vi "ATS_Specs_Selection.vi"(9 "ID":i32, 10 "Device":i32=-1, 11 "ATS_Spec_Selector":T4) -> (0 "Disabled_Item":i32[](array[numeric]), 1 "Possible_Item":string[](array[string]), 2 "All_Item":string[](array[string]), 3 "Selection":string, 4 "Other":cluster{"ValueName":string, "Value":u32}, 5 "Specifications":T5={"ClckSource"={"Internal"=FALSE, "External"=FALSE, "Medium Ext."=FALSE, "Slow Ext."=FALSE, "Ext. AC"=FALSE, "Ext. DC"=FALSE, "Ext. (PLL)"=FALSE}, "ClckRate"={"1 kS/s"=FALSE, "2 kS/s"=FALSE, "5 kS/s"=FALSE, "10 kS/s"=FALSE, "20 kS/s"=FALSE, "50 kS/s"=FALSE, "100 kS/s"=FALSE, "200 kS/s"=FALSE, "500 kS/s"=FALSE, "1 MS/s"=FALSE, "2 MS/s"=FALSE, "5 MS/s"=FALSE, "10 MS/s"=FALSE, "20 MS/s"=FALSE, "25 MS/s"=FALSE, "50 MS/s"=FALSE, "100 MS/s"=FALSE, "125 MS/s"=FALSE, "160 MS/s"=FALSE, "180 MS/s"=FALSE, "200 MS/s"=FALSE, "250 MS/s"=FALSE, "500 MS/s"=FALSE, "1 GS/s"=FALSE}, "ClckEdge"={"Rising"=FALSE, "Falling"=FALSE}, "InputCoupling"={"AC"=FALSE, "DC"=FALSE}, "InputRange"={"20mV"=FALSE, "40mV"=FALSE, "50mV"=FALSE, "80mV"=FALSE, "100mV"=FALSE, "200mV"=FALSE, "400mV"=FALSE, "500mV"=FALSE, "800mV"=FALSE, "1 V"=FALSE, "2 V"=FALSE, "4 V"=FALSE, "5 V"=FALSE, "8 V"=FALSE, "10 V"=FALSE, "16 V"=FALSE, "20 V"=FALSE, "40 V"=FALSE, "HiFi"=FALSE, "1.25 V"=FALSE}, "Impedance"={"1M ohms"=FALSE, "50 ohms"=FALSE, "300 ohms"=FALSE}, "Bandwidth"={"Full"=FALSE, "Reduce"=FALSE}, "RangeLim(50)"="", "AsyncDMA"={"OnBoard"=FALSE, "FPGA"=FALSE}, "Memory"={"VerifMem"=FALSE, "HighMem"=FALSE, "Combine"=FALSE, "HighRecord"=FALSE}, "ExtTrigCoupling"={"AC"=FALSE, "DC"=FALSE}, "ExtTrigRange"={"1 V"=FALSE, "5 V"=FALSE, "\nTTL"=FALSE}, "AUX_IO_Trig"={"Trig_Out"=FALSE, "Trig_In"=FALSE}, "AUX_IO_Slope"={"Rising"=FALSE, "Falling"=FALSE}, "MaxPretrig"={"MEM"=0, "FIFO"=0}, "AUX_I/O_Trig"={"OUT_Trigger"=FALSE, "OUT_PACER"=FALSE, "OUT_BUSY"=FALSE, "OUT_CLOCK"=FALSE, "OUT_RESERVED"=FALSE, "OUT_CAPTURE_ALMOST_DONE"=FALSE, "OUT_AUXILIARY"=FALSE, "OUT_SERIAL_DATA"=FALSE, "IN_TRIGGER_ENABLE"=FALSE, "IN_DIGITAL_TRIGGER"=FALSE, "IN_GATE"=FALSE, "IN_CAPTURE_ON_DEMAND"=FALSE, "IN_RESET_TIMESTAMP"=FALSE, "IN_SLOW_EXTERNAL_CLOCK"=FALSE, "INPUT_AUXILIARY"=FALSE, "INPUT_SERIAL_DATA"=FALSE}, "ChannelsPerBoard"=2}, 7 "Device_Name":string)   [LabVIEW 2015]
doc: "_____AlazarTech, Scope_____\n\nExtract the Selected Specifications of the ID Board and create a text array of All, Possible and Disable item.\n\nIf Device = -1 than use the ID input otherwise select the device.\n\nOutput:\n- Selection: option read\n-All_Item: all specifications array\n-Possible_Item: available specification array\n-Disabled_Item: array of item number which are not available."
uses:
  ATS_ctl/ATS_Global_Specs_Ctrl.ctl
  ATS_ctl/ATS_Spec_Selector.ctl
  ATS_ctl/ATS_TriggerEngine_4Ch.ctl
  ATS_ctl/ATS_TriggerSource_4Ch.ctl
  ATS_ctl/TriggerEngine.ctl
  ATS_ctl/ATS_Global_Ctrl.ctl
  ATS_ctl/ATS_Cards_GBL.vi
panel:
  in  "TrigEngine":T1
  in  "TriggerEngine_4Ch":T2
  out "Device_ID":string
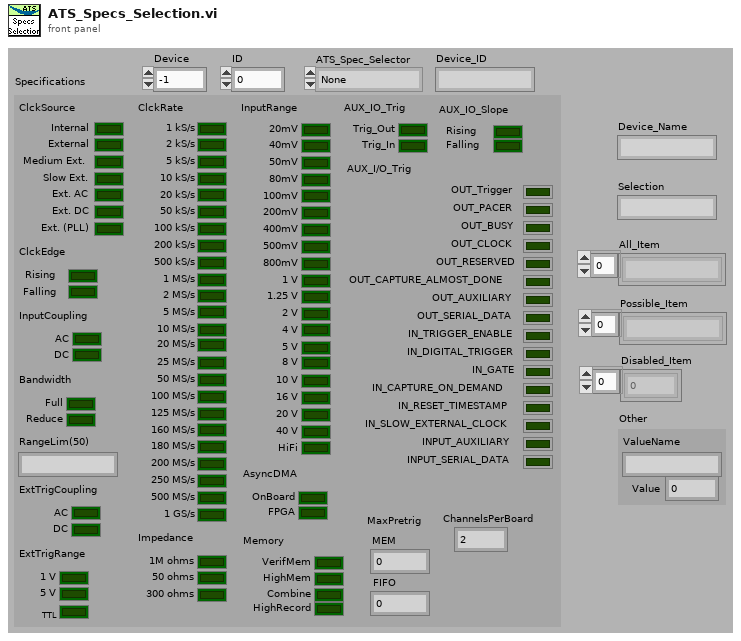
[diagram p1: front panel]
types:
  T1 = typedef "TriggerEngine.ctl" = cluster{"Source":enum32{"Chan_A", "Chan_B", "External", "Disable"}, "Slope":enum32{"Positive", "Negative"}, "Level":u32}
  T2 = typedef "ATS_TriggerEngine_4Ch.ctl" = cluster{"Source":T3, "Slope":enum32{"Positive", "Negative"}, "Level":u32}
  T3 = typedef "ATS_TriggerSource_4Ch.ctl" = enum32{"Chan_A", "Chan_B", "External", "Disable", "Chan_C", "Chan_D"}
  T4 = typedef "ATS_Spec_Selector.ctl" = enum16{"None", "ClckSource", "ClckEdge", "ClckRate", "InputRange", "InputCoupling", "Impedance", "Bandwidth", "AsyncDMA", "Memory", "ExtTrigCoupling", "ExtTrigRange", "AUX_IO_Trig", "AUX_IO_Slope", "Trigger_Source"}
  T5 = typedef "ATS_Global_Specs_Ctrl.ctl" = cluster{"ClckSource":cluster{"Internal":bool, "External":bool, "Medium Ext.":bool, "Slow Ext.":bool, "Ext. AC":bool, "Ext. DC":bool, "Ext. (PLL)":bool}, "ClckRate":cluster{"1 kS/s":bool, "2 kS/s":bool, "5 kS/s":bool, "10 kS/s":bool, "20 kS/s":bool, "50 kS/s":bool, "100 kS/s":bool, "200 kS/s":bool, "500 kS/s":bool, "1 MS/s":bool, "2 MS/s":bool, "5 MS/s":bool, "10 MS/s":bool, "20 MS/s":bool, "25 MS/s":bool, "50 MS/s":bool, "100 MS/s":bool, "125 MS/s":bool, "160 MS/s":bool, "180 MS/s":bool, "200 MS/s":bool, "250 MS/s":bool, "500 MS/s":bool, "1 GS/s":bool}, "ClckEdge":cluster{"Rising":bool, "Falling":bool}, "InputCoupling":cluster{"AC":bool, "DC":bool}, "InputRange":cluster{"20mV":bool, "40mV":bool, "50mV":bool, "80mV":bool, "100mV":bool, "200mV":bool, "400mV":bool, "500mV":bool, "800mV":bool, "1 V":bool, "2 V":bool, "4 V":bool, "5 V":bool, "8 V":bool, "10 V":bool, "16 V":bool, "20 V":bool, "40 V":bool, "HiFi":bool, "1.25 V":bool}, "Impedance":cluster{"1M ohms":bool, "50 ohms":bool, "300 ohms":bool}, "Bandwidth":cluster{"Full":bool, "Reduce":bool}, "RangeLim(50)":string, "AsyncDMA":cluster{"OnBoard":bool, "FPGA":bool}, "Memory":cluster{"VerifMem":bool, "HighMem":bool, "Combine":bool, "HighRecord":bool}, "ExtTrigCoupling":cluster{"AC":bool, "DC":bool}, "ExtTrigRange":cluster{"1 V":bool, "5 V":bool, "\nTTL":bool}, "AUX_IO_Trig":cluster{"Trig_Out":bool, "Trig_In":bool}, "AUX_IO_Slope":cluster{"Rising":bool, "Falling":bool}, "MaxPretrig":cluster{"MEM":u32, "FIFO":u32}, "AUX_I/O_Trig":cluster{"OUT_Trigger":bool, "OUT_PACER":bool, "OUT_BUSY":bool, "OUT_CLOCK":bool, "OUT_RESERVED":bool, "OUT_CAPTURE_ALMOST_DONE":bool, "OUT_AUXILIARY":bool, "OUT_SERIAL_DATA":bool, "IN_TRIGGER_ENABLE":bool, "IN_DIGITAL_TRIGGER":bool, "IN_GATE":bool, "IN_CAPTURE_ON_DEMAND":bool, "IN_RESET_TIMESTAMP":bool, "IN_SLOW_EXTERNAL_CLOCK":bool, "INPUT_AUXILIARY":bool, "INPUT_SERIAL_DATA":bool}, "ChannelsPerBoard":u8}
  T6 = typedef "ATS_Global_Ctrl.ctl" = enum16{"Init_Device", "Clear_ALL", "Set", "Get"}
  T7 = typedef "Device_Info.ctl" = cluster{"Handle":u32, "Board":string, "CPLD":string, "MemorySize":u32, "SampleSize":u8, "ID":i32, "High_Memory":bool, "Chan/Board":u8}
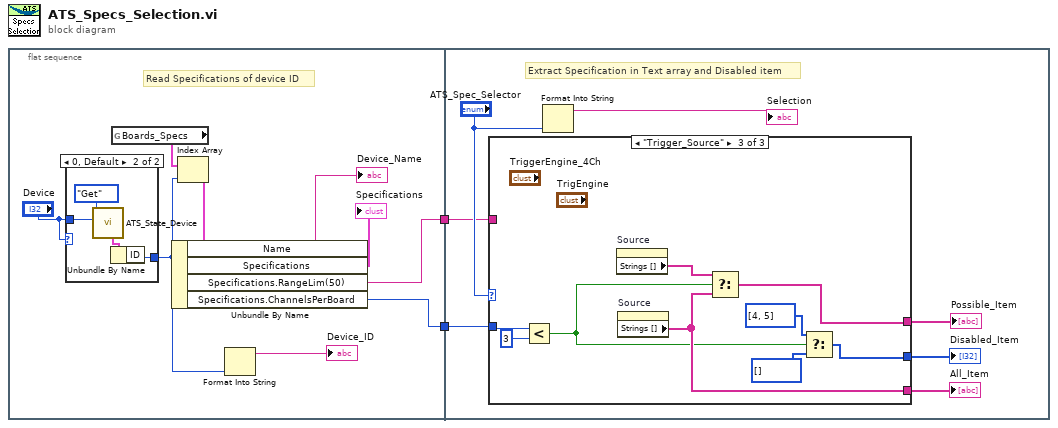
[diagram p0: block diagram]
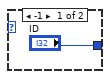
[diagram p2: hidden frame]
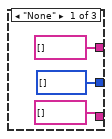
[diagram p3: hidden frame]
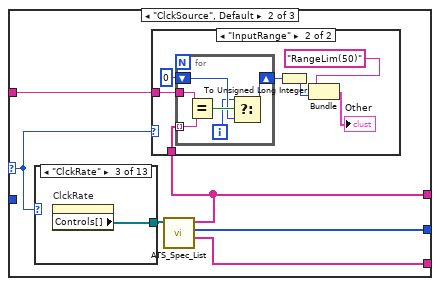
[diagram p4: hidden frame]
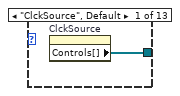
[diagram p6: hidden frame]
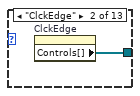
[diagram p7: hidden frame]
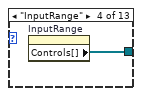
[diagram p8: hidden frame]
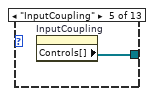
[diagram p9: hidden frame]
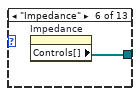
[diagram p10: hidden frame]
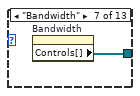
[diagram p11: hidden frame]
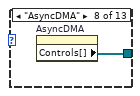
[diagram p12: hidden frame]
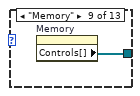
[diagram p13: hidden frame]
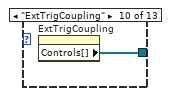
[diagram p14: hidden frame]
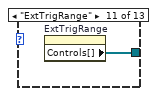
[diagram p15: hidden frame]
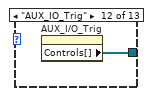
[diagram p16: hidden frame]
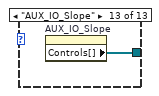
[diagram p17: hidden frame]
diagram:
  n1 = flat-sequence {
    tunnel: [w7] -> w2
    tunnel: [w3] -> w1
    tunnel: w2 -> [w21]
    tunnel: w1 -> [w17]
    frame #0 {
      # "Read Specifications of device ID"
      n2 = case shown="0, Default" "Device" {
        tunnel: "Device" -> [_ w15]
        tunnel: ["ID" w13] -> w5
        frame -1 {
        }
        frame 0, Default {
          n3 = call "ATS_State_Device.vi"("DeviceIn"=w15, "ATS_GBL_Ctrl"=ATS_Global_Ctrl."Get") -> ("DevInfo_Out"=w14:T7)  [unwired: 4 in, 5 out]
          n4 = Unbundle By Name(w14) -> ("ID"=w13:i32)
        }
      }
      n5 = global read "ATS_Cards_GBL.vi" "Boards_Specs"() -> (w4:cluster{"Name":string, "Specifications":T5}[])
      n6 = Index Array(array=w4, index=w5) -> (element=w11:cluster{"Name":string, "Specifications":T5})
      n7 = Unbundle By Name(w11) -> ("Name"=→"Device_Name":string, "Specifications"=→"Specifications":T5, "Specifications.RangeLim(50)"=w7:string, "Specifications.ChannelsPerBoard"=w3:u8)
      n8 = Format Into String(w5) -> (resulting string=→"Device_ID":string)  [unwired: 3 in, 1 out]
    }
    frame #1 {
      # "Extract Specification in Text array and Disabled item"
      n9 = case shown="\"Trigger_Source\"" "ATS_Spec_Selector" {
        selector: "ATS_Spec_Selector" -> [_ w30 _]
        tunnel: w21 -> [_ w31 _]
        tunnel: [string[] [] ("Selected_Item") w29 w65] -> w20
        tunnel: [i32[] [] ("Disabled Items") w28 w59] -> w19
        tunnel: [string[] [] ("Complete_List") w27 w64] -> w18
        tunnel: w17 -> [_ _ w67]
        frame "None" {
        }
        frame "ClckSource", Default {
          n10 = case shown="\"ClckRate\"" w30 {
            tunnel: [w46 w47 w48 w49 w50 w51 w52 w53 w54 w55 w56 w57 w58] -> w32
            frame "ClckSource", Default {
              n11 = property on="ClckSource" class="Clust (strict)"() -> ("Controls[]"=w46:refnum<vi>[])  [unwired: 2 in, 2 out]
            }
            frame "ClckEdge" {
              n12 = property on="ClckEdge" class="Clust (strict)"() -> ("Controls[]"=w47:refnum<vi>[])  [unwired: 2 in, 2 out]
            }
            frame "ClckRate" {
              n13 = property on="ClckRate" class="Clust (strict)"() -> ("Controls[]"=w48:refnum<vi>[])  [unwired: 2 in, 2 out]
            }
            frame "InputRange" {
              n14 = property on="InputRange" class="Clust (strict)"() -> ("Controls[]"=w49:refnum<vi>[])  [unwired: 2 in, 2 out]
            }
            frame "InputCoupling" {
              n15 = property on="InputCoupling" class="Clust (strict)"() -> ("Controls[]"=w50:refnum<vi>[])  [unwired: 2 in, 2 out]
            }
            frame "Impedance" {
              n16 = property on="Impedance" class="Clust (strict)"() -> ("Controls[]"=w51:refnum<vi>[])  [unwired: 2 in, 2 out]
            }
            frame "Bandwidth" {
              n17 = property on="Bandwidth" class="Clust (strict)"() -> ("Controls[]"=w52:refnum<vi>[])  [unwired: 2 in, 2 out]
            }
            frame "AsyncDMA" {
              n18 = property on="AsyncDMA" class="Clust (strict)"() -> ("Controls[]"=w53:refnum<vi>[])  [unwired: 2 in, 2 out]
            }
            frame "Memory" {
              n19 = property on="Memory" class="Clust (strict)"() -> ("Controls[]"=w54:refnum<vi>[])  [unwired: 2 in, 2 out]
            }
            frame "ExtTrigCoupling" {
              n20 = property on="ExtTrigCoupling" class="Clust (strict)"() -> ("Controls[]"=w55:refnum<vi>[])  [unwired: 2 in, 2 out]
            }
            frame "ExtTrigRange" {
              n21 = property on="ExtTrigRange" class="Clust (strict)"() -> ("Controls[]"=w56:refnum<vi>[])  [unwired: 2 in, 2 out]
            }
            frame "AUX_IO_Trig" {
              n22 = property on="AUX_I/O_Trig" class="Clust (strict)"() -> ("Controls[]"=w57:refnum<vi>[])  [unwired: 2 in, 2 out]
            }
            frame "AUX_IO_Slope" {
              n23 = property on="AUX_IO_Slope" class="Clust (strict)"() -> ("Controls[]"=w58:refnum<vi>[])  [unwired: 2 in, 2 out]
            }
          }
          n24 = call "ATS_Spec_List.vi"("Controls[]"=w32) -> ("Complete_List"=w27:string[], "Disabled Items"=w28:i32[], "Selected_Item"=w29:string[])  [unwired: 8 in]
          n25 = case shown="\"InputRange\"" w30 {
            tunnel: w29 -> [_ w37]
            tunnel: w31 -> [_ w36]
            frame "None", Default {
            }
            frame "InputRange" {
              n26 = for {
                tunnel: w37 -> [w44] mode=indexing
                tunnel: w36 -> [w45]
                shift-right: [w42] -> w38
                shift-left: 0 ("Numeric") -> [w41]
                i -> [w40]
                n27 = Equal?(x=w45, y=w44) -> (x = y?=w43:bool)
                n28 = Select(t=w40, s=w43, f=w41) -> (s? t:f=w42:i32)
              }
              n29 = To Unsigned Long Integer(number=w38) -> (unsigned 32bit integer=w35:u32)
              n30 = Bundle("RangeLim(50)", w35) -> (→"Other":cluster{string, u32})  [unwired: 1 in]
            }
          }
        }
        frame "Trigger_Source" {
          n31 = Less?(x=w67, y=u8 3) -> (x < y?=w62:bool)
          n32 = property on="Source" class="Enum (strict)"() -> ("Strings []"=w63:string[])  [unwired: 2 in, 2 out]
          n33 = property on="Source" class="Enum (strict)"() -> ("Strings []"=w64:string[])  [unwired: 2 in, 2 out]
          n34 = Select(t=w63, s=w62, f=w64) -> (s? t:f=w65:string[])
          n35 = Select(t=i32[] [4, 5] ("Disabled Items"), s=w62, f=i32[] [] ("Disabled Items")) -> (s? t:f=w59:i32[])
        }
      }
      "Disabled_Item" <- w19
      "All_Item" <- w18
      "Possible_Item" <- w20
      n36 = Format Into String("ATS_Spec_Selector") -> (resulting string=→"Selection":string)  [unwired: 3 in, 1 out]
    }
  }
